vi "LIA DFD Decimation.vi"(7 "filter in":T1 {"mSRate_QSettings"."source" items=["Coef a/k"=0, "Coef b/v"=7, "Input"=1, "Output"=2, "Multiplicand"=3, "Product"=4, "Sum"=5, "Delay"=6, "Gain"=8]}, 9 "decimation base":i32=2, 10 "decimate by x times":i32=2, 11 "data in":cdb[](array[numeric])) -> (2 "total decimation":dbl, 3 "decimated data":cdb[](array[numeric]))   [LabVIEW 2018]
uses:
  <vilib>/addons/Digital Filter Design/_Objects.llb/DFD Filter Obj.ctl
  <vilib>/addons/Digital Filter Design/_Objects.llb/DFD Filter Coef.ctl
  <vilib>/addons/Digital Filter Design/_Objects.llb/DFD Filter Structure Type Selector.ctl
  <vilib>/addons/Digital Filter Design/_Objects.llb/dfd_Internal Quantization Settings.ctl
  <vilib>/addons/Digital Filter Design/_Objects.llb/dfd_Internal Quantization Srcs.ctl
  <vilib>/addons/Digital Filter Design/_Objects.llb/DFD Coef Norm Type.ctl
  <vilib>/addons/Digital Filter Design/NI_DigFilterLicensed.lvlib
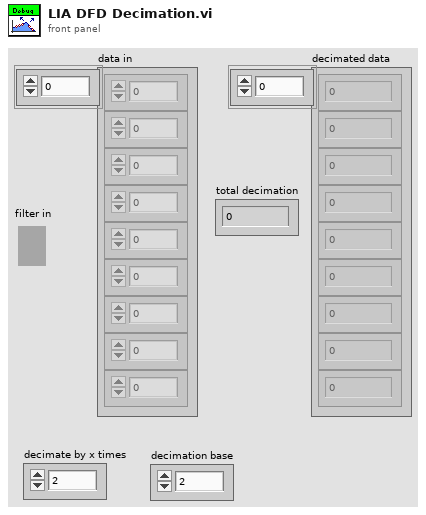
[diagram p1: front panel]
types:
  T1 = typedef "NI_DigFilterLicensed.lvlib/DFD Filter Obj.ctl" = cluster{"mSRate_Fs":dbl, "mSRate_Version":string, "mSRate_Comments":string, "mSRate_OrgCoef":T2, "mSRate_CurCoef":T2, "mSRate_Quantized?":bool, "mSRate_QCoef":T2, "mSRate_QSettings":T4[], "mSRate_Order":i32, "mSRate_Scaling":cluster{"mSRate_ScaleByPowerOf2?":bool, "mSRate_ScaleType":T6}}
  T2 = typedef "NI_DigFilterLicensed.lvlib/DFD Filter Coef.ctl" = cluster{"type":T3, "gain":dbl, "coef a (k)":dbl[], "coef b (v)":dbl[]}
  T3 = typedef "NI_DigFilterLicensed.lvlib/DFD Filter Structure Type Selector.ctl" = enum16{"Undefined", "FIR Direct Form", "FIR Direct Form Transposed", "FIR Symmetric", "FIR Antisymmetric", "IIR Direct Form I", "IIR Direct Form I Transposed", "IIR Direct Form II", "IIR Direct Form II Transposed", "IIR Cascaded Second Order Sections Form I", "IIR Cascaded Second Order Sections Form I Transposed", "IIR Cascaded Second Order Sections Form II", "IIR Cascaded Second Order Sections Form II Transposed", "Lattice Allpass (basic sections)", "Lattice Allpass (one multiplier sections)", "Lattice Allpass (normalized sections)", "Lattice AR (basic sections)", "Lattice AR (one multiplier sections)", "Lattice AR (normalized sections)", "Lattice MA (minimum phase)", "Lattice MA (maximum phase)", "Lattice ARMA (basic sections)", "Lattice ARMA (one multiplier sections)", "Lattice ARMA (normalized sections)"}
  T4 = typedef "NI_DigFilterLicensed.lvlib/dfd_Internal Quantization Settings.ctl" = cluster{"source":T5, "wl":i16, "iwl":i16, "overflow mode":enum16{"Saturation", "Wrap"}, "rounding mode":enum16{"Nearest", "Truncation"}, "signed?":bool}
  T5 = typedef "NI_DigFilterLicensed.lvlib/dfd_Internal Quantization Srcs.ctl" = u16
  T6 = typedef "NI_DigFilterLicensed.lvlib/DFD Coef Norm Type.ctl" = enum16{"No Norm", "Time Domain 1-Norm", "Time Domain 2-Norm", "Time Domain Inf-Norm"}
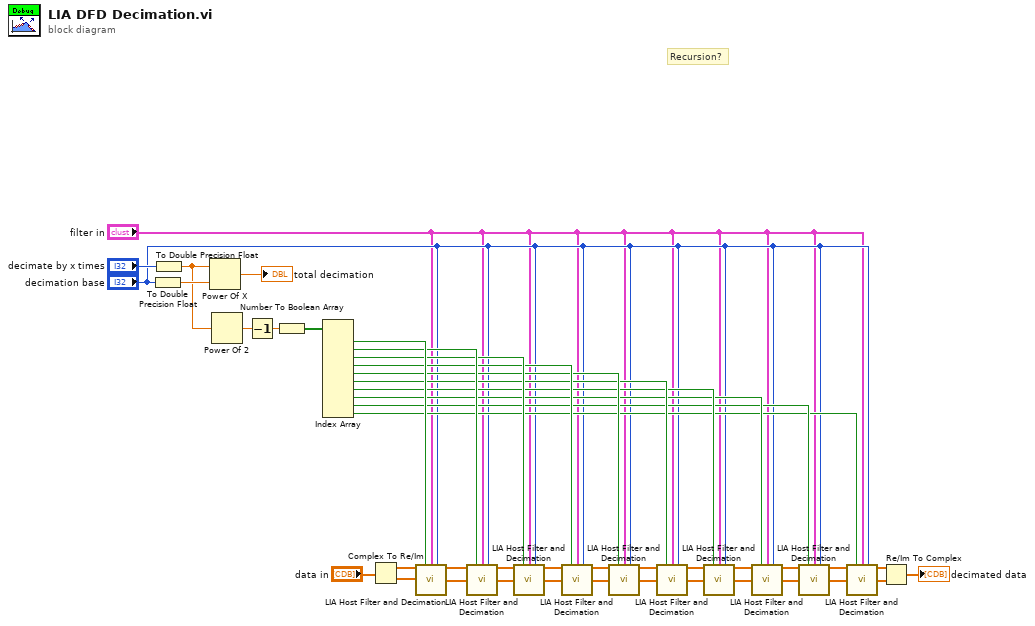
[diagram p0: block diagram]
diagram:
  # "Recursion?"
  n1 = To Double Precision Float(number="decimation base") -> (double precision float=w40:dbl)
  n2 = To Double Precision Float(number="decimate by x times") -> (double precision float=w38:dbl)
  n3 = Power Of X(1:w40, 2:w38) -> (0:→"total decimation":dbl)
  n4 = Power Of 2(x=w38) -> (2^x=w37:dbl)
  n5 = Decrement(x=w37) -> (x-1=w36:dbl)
  n6 = Number To Boolean Array(number=w36) -> (Boolean array=w35:bool[])
  n7 = Index Array(array=w35) -> (element #1=w32:bool, element #2=w21:bool, element #3=w20:bool, element #4=w19:bool, element #5=w18:bool, element #6=w17:bool, element #7=w16:bool, element #8=w5:bool, element #9=w4:bool, element #10=w3:bool)  [unwired: 10 in]
  n8 = Complex To Re/Im(x + iy="data in") -> (x=w34:dbl[], y=w33:dbl[])
  n9 = call "LIA Host Filter and Decimation.vi"("I in"=w34, "Enable?"=w32, "filter in in"="filter in", "decimation base in"="decimation base", "Q in"=w33) -> ("Decimated I"=w31:dbl[], "Decimated Q"=w15:dbl[])  [unwired: 9 in]
  n10 = call "LIA Host Filter and Decimation.vi"("I in"=w31, "Enable?"=w21, "filter in in"="filter in", "decimation base in"="decimation base", "Q in"=w15) -> ("Decimated I"=w30:dbl[], "Decimated Q"=w14:dbl[])  [unwired: 9 in]
  n11 = call "LIA Host Filter and Decimation.vi"("I in"=w30, "Enable?"=w20, "filter in in"="filter in", "decimation base in"="decimation base", "Q in"=w14) -> ("Decimated I"=w29:dbl[], "Decimated Q"=w13:dbl[])  [unwired: 9 in]
  n12 = call "LIA Host Filter and Decimation.vi"("I in"=w29, "Enable?"=w19, "filter in in"="filter in", "decimation base in"="decimation base", "Q in"=w13) -> ("Decimated I"=w28:dbl[], "Decimated Q"=w12:dbl[])  [unwired: 9 in]
  n13 = call "LIA Host Filter and Decimation.vi"("I in"=w28, "Enable?"=w18, "filter in in"="filter in", "decimation base in"="decimation base", "Q in"=w12) -> ("Decimated I"=w27:dbl[], "Decimated Q"=w11:dbl[])  [unwired: 9 in]
  n14 = call "LIA Host Filter and Decimation.vi"("I in"=w27, "Enable?"=w17, "filter in in"="filter in", "decimation base in"="decimation base", "Q in"=w11) -> ("Decimated I"=w24:dbl[], "Decimated Q"=w10:dbl[])  [unwired: 9 in]
  n15 = call "LIA Host Filter and Decimation.vi"("I in"=w24, "Enable?"=w16, "filter in in"="filter in", "decimation base in"="decimation base", "Q in"=w10) -> ("Decimated I"=w26:dbl[], "Decimated Q"=w9:dbl[])  [unwired: 9 in]
  n16 = call "LIA Host Filter and Decimation.vi"("I in"=w26, "Enable?"=w5, "filter in in"="filter in", "decimation base in"="decimation base", "Q in"=w9) -> ("Decimated I"=w23:dbl[], "Decimated Q"=w8:dbl[])  [unwired: 9 in]
  n17 = call "LIA Host Filter and Decimation.vi"("I in"=w23, "Enable?"=w4, "filter in in"="filter in", "decimation base in"="decimation base", "Q in"=w8) -> ("Decimated I"=w22:dbl[], "Decimated Q"=w7:dbl[])  [unwired: 9 in]
  n18 = call "LIA Host Filter and Decimation.vi"("I in"=w22, "Enable?"=w3, "filter in in"="filter in", "decimation base in"="decimation base", "Q in"=w7) -> ("Decimated I"=w25:dbl[], "Decimated Q"=w6:dbl[])  [unwired: 9 in]
  n19 = Re/Im To Complex(1:w6, 2:w25) -> (0:→"decimated data":cdb[])
